vi "LVPortVariantArrayTo1DArrayOfRealFast.vi"(11 "Variant Real Array":variant) -> (1 "N dims":u32, 2 "Size(s)":u32[](array[numeric]), 3 "1D Array":dbl[](array[numeric]))   [LabVIEW 2017]
panel:
  in  "Array Type":dbl
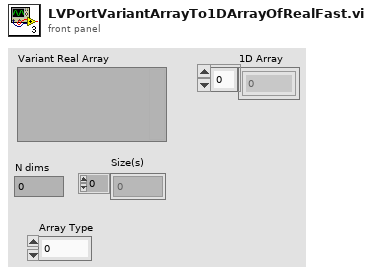
[diagram p1: front panel]
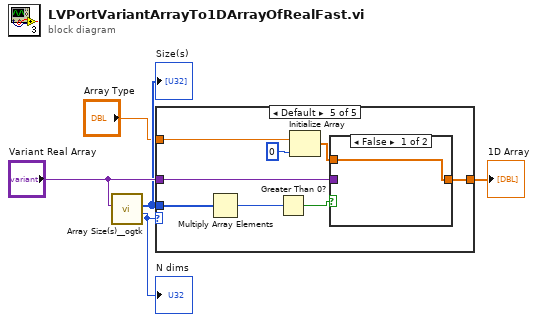
[diagram p0: block diagram]
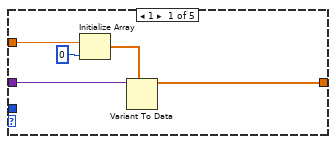
[diagram p2: hidden frame]
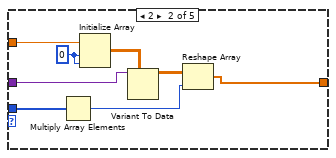
[diagram p3: hidden frame]
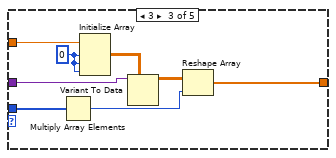
[diagram p4: hidden frame]
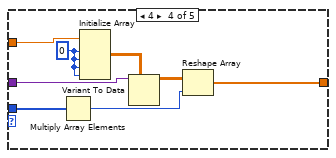
[diagram p5: hidden frame]
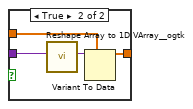
[diagram p6: hidden frame]
diagram:
  n1 = call <userlib>:"Array Size(s)__ogtk.vi"("Array"="Variant Real Array") -> ("N dims"=w5:u32, "Size(s)"=w3:u32[])  [unwired: 8 in, 1 out]
  "Size(s)" <- w3
  "N dims" <- w5
  n2 = case shown="Default" w5 {
    tunnel: [w10 w14 w22 w30 w35] -> w1
    tunnel: "Variant Real Array" -> [w9 w18 w26 w34 w39]
    tunnel: w3 -> [_ w16 w24 w32 w42]
    tunnel: "Array Type" -> [w7 w13 w21 w29 w38]
    frame 1 {
      n3 = Initialize Array(w7, 0 ("dimension size")) -> (w6:dbl[])
      n4 = Variant To Data(type=w6, Variant=w9) -> (data=w10:dbl[])  [unwired: 1 in, 1 out]
    }
    frame 2 {
      w12 = 0 ("dimension size")
      n5 = Multiply Array Elements(1:w16) -> (0:w15:u32)
      n6 = Initialize Array(w13, w12, w12) -> (w11:dbl[][])
      n7 = Variant To Data(type=w11, Variant=w18) -> (data=w17:dbl[][])  [unwired: 1 in, 1 out]
      n8 = Reshape Array(w17, w15) -> (w14:dbl[])
    }
    frame 3 {
      w19 = 0 ("dimension size")
      n9 = Multiply Array Elements(1:w24) -> (0:w23:u32)
      n10 = Initialize Array(w21, w19, w19, w19) -> (w20:dbl[][][])
      n11 = Variant To Data(type=w20, Variant=w26) -> (data=w25:dbl[][][])  [unwired: 1 in, 1 out]
      n12 = Reshape Array(w25, w23) -> (w22:dbl[])
    }
    frame 4 {
      w27 = 0 ("dimension size")
      n13 = Multiply Array Elements(1:w32) -> (0:w31:u32)
      n14 = Initialize Array(w29, w27, w27, w27, w27) -> (w28:dbl[][][][])
      n15 = Variant To Data(type=w28, Variant=w34) -> (data=w33:dbl[][][][])  [unwired: 1 in, 1 out]
      n16 = Reshape Array(w33, w31) -> (w30:dbl[])
    }
    frame Default {
      n17 = Multiply Array Elements(1:w42) -> (0:w41:u32)
      n18 = Greater Than 0?(x=w41) -> (x > 0?=w40:bool)
      n19 = Initialize Array(w38, 0 ("dimension size")) -> (w36:dbl[])
      n20 = case shown="False" w40 {
        tunnel: [w43 w46] -> w35
        tunnel: w39 -> [_ w47]
        tunnel: w36 -> [w43 w44]
        frame False {
        }
        frame True {
          n21 = call <userlib>:"Reshape Array to 1D VArray__ogtk.vi"("MultiD Array"=w47) -> ("1D VArray"=w45:variant)  [unwired: 8 in, 2 out]
          n22 = Variant To Data(type=w44, Variant=w45) -> (data=w46:dbl[])  [unwired: 1 in, 1 out]
        }
      }
    }
  }
  "1D Array" <- w1
